vi "Stop Core.vi"(10 "final error code":i32, 11 "TestActor in":refnum<class "TestActor.lvclass">) -> (3 "TestActor out":refnum<class "TestActor.lvclass">)   [LabVIEW 2015, in "TestActor.lvlib" / "TestActor.lvclass"]
doc: "(<B>Filename</B>: Actor Framework.lvlib:Actor.lvclass:Stop Core.vi)\n\nDefines what the actor does before it stops. Use the <B>final error code</B> input to determine whether the actor shut down in response to an error.\n\nBy default, this method does nothing. A descendant class may override it to define behavior, such as shutting down any processes the actor initiated in its override of the Actor Core method."
uses:
  TestActor.lvclass
  TestActor.lvclass/TestActor.ctl
  CSPP_Core/Actors/CS++BaseActor/CS++BaseActor.lvclass
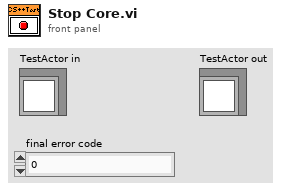
[diagram p1: front panel]
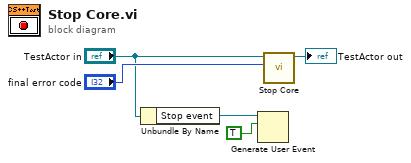
[diagram p0: block diagram]
diagram:
  n1 = Unbundle By Name("TestActor in") -> ("Stop event"=w2:refnum<user-event>)
  n2 = Generate User Event(user event=w2, event data cluster=TRUE) -> ()  [unwired: 2 in, 2 out]
  n3 = call-parent "Stop Core.vi"("final error code"="final error code", "CS++BaseActor in"="TestActor in") -> ("CS++BaseActor out"=→"TestActor out":refnum<class "TestActor.lvclass">)  [unwired: 9 in]
